vi "LoggingUtil.vi"(7 "Enable":bool=TRUE, 8 "Log Item":string, 9 "Queue":refnum<queue>, 11 "Command":enum16{"Log", "Terminate"}(ring)) -> ()   [LabVIEW 2010, in "lib1299.lvlib"]
doc: "This VI serves to log the commands retrieved from various queues (specific queue noted in log file)."
uses:
  lib1299.lvlib
  <userlib>/Common/Queue with Cluster/TYP_Queue Cluster Element.ctl
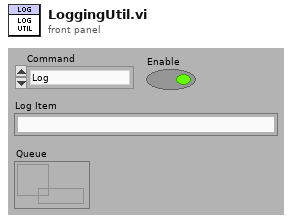
[diagram p1: front panel]
types:
  T1 = enum16{"open", "replace", "create", "open or create", "replace or create", "replace or create with confirmation"}
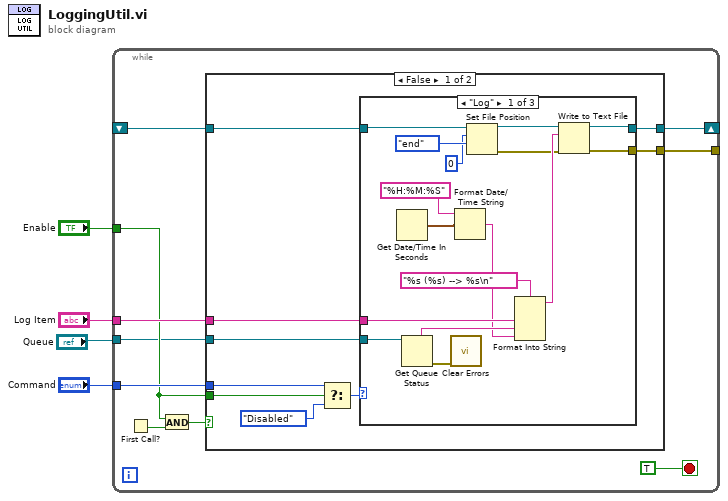
[diagram p0: block diagram]
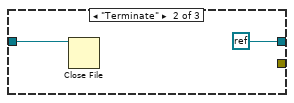
[diagram p2: hidden frame]
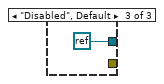
[diagram p3: hidden frame]
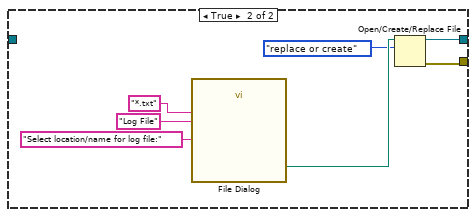
[diagram p4: hidden frame]
diagram:
  n1 = while {
    shift-right: [w13] -> _
    shift-left: _ -> [w12]
    tunnel: "Command" -> [w11]
    tunnel: "Log Item" -> [w10]
    tunnel: "Enable" -> [w7]
    tunnel: "Queue" -> [w6]
    tunnel: [w5] -> _
    stop <- TRUE stop-if-true
    n2 = First Call?() -> (First Call?: T/F=w8:bool)
    n3 = And(x=w7, y=w8) -> (x .and. y?=w9:bool)
    n4 = case shown="False" w9 {
      tunnel: [w22 w48] -> w13
      tunnel: w12 -> [w23 _]
      tunnel: w11 -> [w19 _]
      tunnel: w10 -> [w21 _]
      tunnel: w7 -> [w18 _]
      tunnel: w6 -> [w16 _]
      tunnel: [w15 w44] -> w5
      frame False {
        n5 = Select(t=w19, s=w18, f=enum16{"Log", "Terminate", "Disabled"}."Disabled") -> (s? t:f=w20:enum16{"Log", "Terminate", "Disabled"})
        n6 = case shown="\"Log\"" w20 {
          tunnel: w23 -> [w39 w40 _]
          tunnel: [w35 refnum<k0> refnum refnum<k0> refnum] -> w22
          tunnel: w21 -> [w34 _ _]
          tunnel: w16 -> [w31 _ _]
          tunnel: [w29 _ _] -> w15
          frame "Log" {
            n7 = Get Date/Time In Seconds() -> (seconds since 1Jan1904=w26:timestamp)
            n8 = Get Queue Status(queue=w31) -> (queue name=w30:string, error out=w28:errorcluster)  [unwired: 1 in, 7 out]
            n9 = call <vilib>:"Clear Errors.vi"("error in (no error)"=w28) -> ()  [unwired: 7 out]
            n10 = Format Date/Time String(time format string (%c)="%H:%M:%S", seconds (now)=w26) -> (date/time string=w24:string)  [unwired: 1 in]
            n11 = Set File Position(offset (in bytes) (0)=i64 0, refnum=w39, from (0:start)=enum16{"start", "end", "current"}."end") -> (refnum out=w36:refnum<file>, error out=w27:errorcluster)  [unwired: 1 in]
            n12 = Format Into String(format string="%s (%s) --> %s\n", w34, w30, w24) -> (resulting string=w32:string)  [unwired: 2 in, 1 out]
            n13 = Write to Text File(file (use dialog)=w36, text=w32, error in=w27) -> (refnum out=w35:refnum<file>, error out=w29:errorcluster)  [unwired: 2 out]
          }
          frame "Terminate" {
            n14 = Close File(refnum=w40) -> ()  [unwired: 1 in, 2 out]
          }
          frame "Disabled", Default {
          }
        }
      }
      frame True {
        n15 = call "File Dialog"("prompt"="Select location/name for log file:", "pattern (all files)"="*.txt", "pattern label"="Log File") -> ("selected path"=w49:path)  [unwired: 4 in, 8 out]
        n16 = Open/Create/Replace File(file path (use dialog)=w49, operation (0:open)=T1."replace or create") -> (refnum out=w48:refnum<file>, error out=w44:errorcluster)  [unwired: 4 in, 1 out]
      }
    }
  }
